vi "Try Match Abort.vi"(8 "error in":errorcluster, 10 "Frame Data":u8[](array[numeric]), 11 "SDO Transfer in":refnum<class "SDO Transfer.lvclass">) -> (0 "error out":errorcluster, 2 "Match":bool, 3 "SDO Transfer out":refnum<class "SDO Transfer.lvclass">)   [LabVIEW 2020, in "CANopen.lvlib" / "SDO Manager.lvlib" / "SDO Transfer.lvclass"]
uses:
  SDO Transfer/SDO Transfer.lvclass
  SDO Transfer/SDO Transfer.lvclass/SDO Transfer.ctl
  SDO Transfer/SDO abort code.ctl
  Typedefs/SDO Result.ctl
  SDO Transfer/SDO Transfer Result.ctl
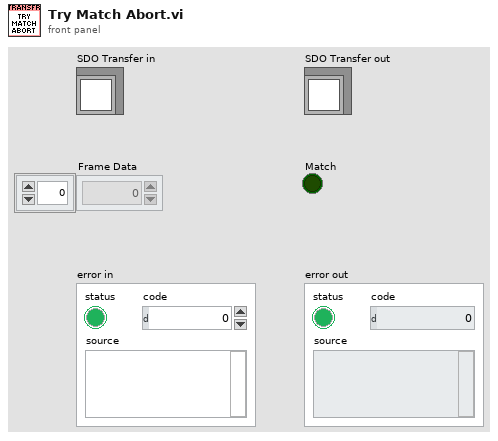
[diagram p1: front panel]
types:
  T1 = typedef "CANopen.lvlib/SDO Manager.lvlib/SDO Transfer.lvclass/SDO Transfer Result.ctl" = cluster{"SDO Result":T2, "Error":errorcluster}
  T2 = typedef "CANopen.lvlib/SDO Manager.lvlib/SDO Transfer.lvclass/SDO Result.ctl" = cluster{"Success":bool, "SDO abort code":cluster{"Null":bool, "Value":T3}, "Data":cluster{"Null":bool, "Data":u8[]}}
  T3 = typedef "CANopen.lvlib/SDO Manager.lvlib/SDO Transfer.lvclass/SDO abort code.ctl" = u32
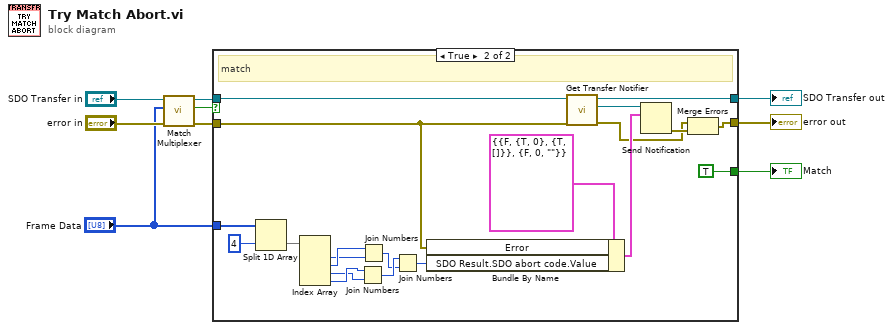
[diagram p0: block diagram]
diagram:
  n1 = call "Match Multiplexer.vi"("error in"="error in", "Frame Data"="Frame Data", "SDO Transfer in"="SDO Transfer in") -> ("error out"=w4:errorcluster, "Match"=w2:bool, "SDO Transfer out"=w3:refnum<class "SDO Transfer.lvclass">)  [unwired: 6 in]
  n2 = case shown="True" w2 {
    tunnel: w4 -> [w11 w17]
    tunnel: w3 -> [w10 w29]
    tunnel: [w10 w27] -> w7
    tunnel: [w11 w16] -> w8
    tunnel: [_ TRUE] -> w9
    tunnel: "Frame Data" -> [_ w13]
    frame False {
      # "no match"
    }
    frame True {
      # "match"
      n3 = Split 1D Array(array=w13, index=4) -> (second subarray=w12:u8[])  [unwired: 1 out]
      n4 = Index Array(array=w12) -> (element #1=w19:u8, element #2=w20:u8, element #3=w21:u8, element #4=w22:u8)  [unwired: 4 in]
      n5 = Join Numbers(hi=w22, lo=w21) -> ((hi.lo)=w31:u16)
      n6 = Join Numbers(hi=w20, lo=w19) -> ((hi.lo)=w30:u16)
      n7 = Join Numbers(hi=w31, lo=w30) -> ((hi.lo)=w25:u32)
      n8 = Bundle By Name(cluster=T1 {"SDO Result"={"Success"=FALSE, "SDO abort code"={"Null"=TRUE, "Value"=0}, "Data"={"Null"=TRUE, "Data"=[]}}, "Error"={"status"=FALSE, "code"=0, "source"=""}} ("SDO Transfer Result"), "Error"=w17, "SDO Result.SDO abort code.Value"=w25) -> (w26:T1)
      n9 = call "Get Transfer Notifier.vi"("error in"=w17, "SDO Transfer in"=w29) -> ("error out"=w15:errorcluster, "SDO Transfer Notifier"=w28:refnum<notifier>, "SDO Transfer out"=w27:refnum<class "SDO Transfer.lvclass">)  [unwired: 7 in]
      n10 = Send Notification(notification=w26, notifier=w28) -> (error out=w24:errorcluster)  [unwired: 1 in, 1 out]
      n11 = Merge Errors(w15, w24) -> (w16:errorcluster)
    }
  }
  "Match" <- w9
  "error out" <- w8
  "SDO Transfer out" <- w7
